vi "kCoerceInt16.vi"(9 "lower":i16, 10 "input":i16, 11 "upper":i16) -> (0 "coerced?":bool, 2 "output":i16)   [LabVIEW 2010, in "KevLib01.lvlib"]
uses:
  KevLib01.lvlib
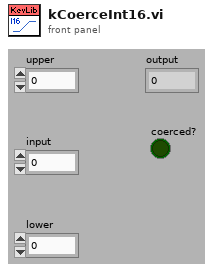
[diagram p1: front panel]
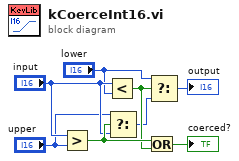
[diagram p0: block diagram]
diagram:
  n1 = Greater?(x="input", y="upper") -> (0:w7:bool)
  n2 = Less?(x="input", y="lower") -> (x < y?=w6:bool)
  n3 = Select(t="upper", s=w7, f="input") -> (s? t:f=w3:i16)
  n4 = Or(x=w7, y=w6) -> (x .or. y?=→"coerced?":bool)
  n5 = Select(t="lower", s=w6, f=w3) -> (s? t:f=→"output":i16)
